vi "Get piezo voltage.vi"(8 "error in (no error)":errorcluster, 11 "COM port in":refnum<visa-resource-name>) -> (0 "error out":errorcluster, 2 "Piezo Voltage":dbl, 3 "COM port out":refnum<visa-resource-name>)   [LabVIEW 2020]
panel:
  out "read buffer":string
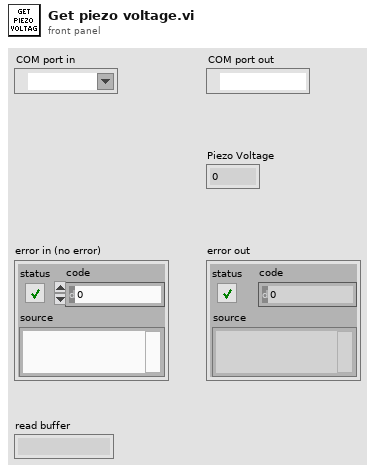
[diagram p1: front panel]
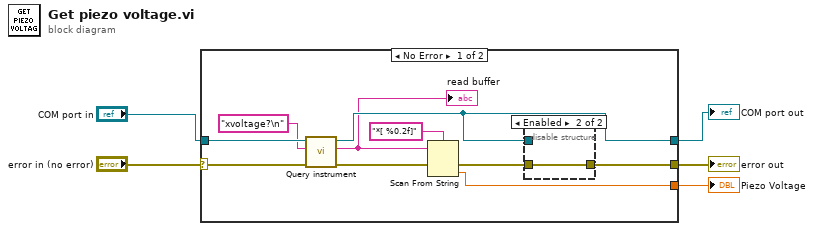
[diagram p0: block diagram]
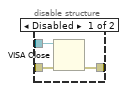
[diagram p2: hidden frame]
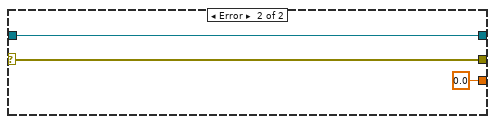
[diagram p3: hidden frame]
diagram:
  n1 = case shown="No Error" "error in (no error)" {
    selector: "error in (no error)" -> [w15 w22]
    tunnel: [w11 w22] -> w4
    tunnel: "COM port in" -> [w14 w21]
    tunnel: [w10 w21] -> w2
    tunnel: [w7 0.0] -> w1
    frame No Error {
      n2 = call "Query instrument.vi"("error in (no error)"=w15, "Command"="xvoltage?\n", "COM port in"=w14) -> ("error out"=w12:errorcluster, "read buffer"=w6:string, "COM port out"=w10:refnum<visa-resource-name>)  [unwired: 6 in]
      "read buffer" <- w6
      n3 = Scan From String(format string="*[ %0.2f]", input string=w6, error in=w12) -> (error out=w9:errorcluster, output 1=w7:dbl)  [unwired: 2 in, 2 out]
      n4 = disable-structure shown="Enabled" {
        disable-tunnel: [w18 w19] -> w11
        disable-tunnel: w10 -> [w17 _]
        disable-tunnel: w9 -> [w16 w19]
        frame Disabled {
          n5 = VISA Close(VISA resource name=w17, error in (no error)=w16) -> (error out=w18:errorcluster)
        }
        frame Enabled {
        }
      }
    }
    frame Error {
    }
  }
  "error out" <- w4
  "COM port out" <- w2
  "Piezo Voltage" <- w1
